vi "Read Publish Camera Settings Msg.vi"(8 "error in (no error)":errorcluster, 11 "Camera Actor in":refnum<class "Camera Actor.lvclass">) -> (0 "error out":errorcluster, 2 "Camera Actor.lvlib:Publish Camera Settings Msg.lvclass":refnum<class "Publish Camera Settings Msg.lvclass">, 3 "Camera Actor out":refnum<class "Camera Actor.lvclass">)   [LabVIEW 2020, in "Camera Actor.lvlib" / "Camera Actor.lvclass"]
uses:
  Camera Actor.lvclass
  Camera Actor Messages/Publish Camera Settings Msg/Publish Camera Settings Msg.lvclass
  Camera Actor.lvclass/Camera Actor.ctl
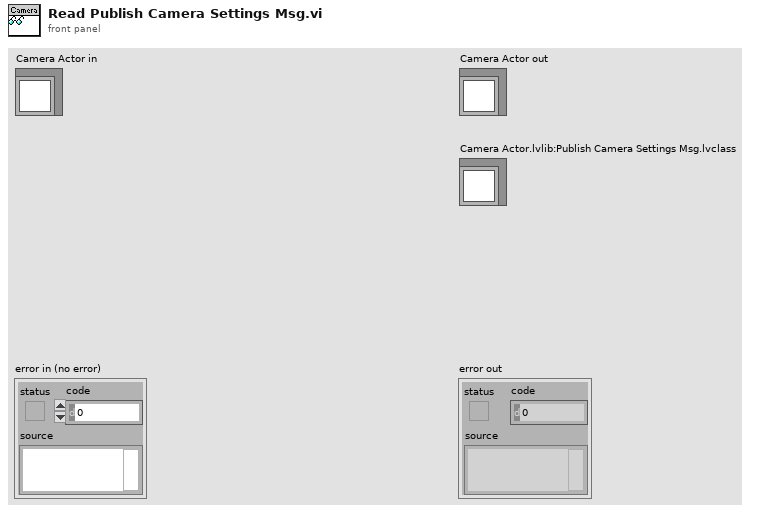
[diagram p1: front panel]
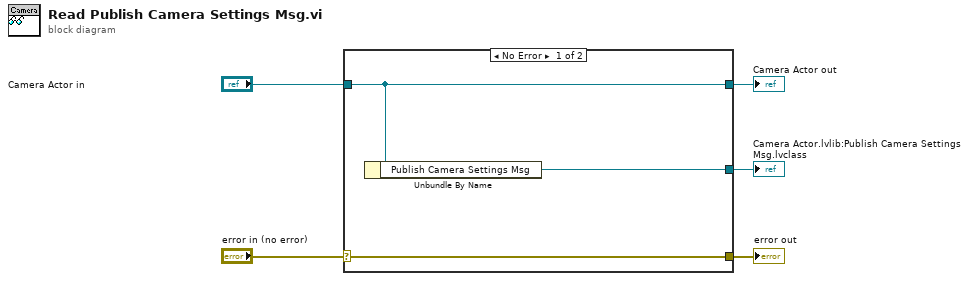
[diagram p0: block diagram]
diagram:
  n1 = case shown="No Error" "error in (no error)" {
    selector: "error in (no error)" -> [w8 w9]
    tunnel: [w8 w9] -> w4
    tunnel: [w7 w10] -> w2
    tunnel: "Camera Actor in" -> [w7 w10]
    tunnel: [w6 _] -> w1
    frame No Error {
      n2 = Unbundle By Name(w7) -> ("Publish Camera Settings Msg"=w6:refnum<class "Publish Camera Settings Msg.lvclass">)
    }
    frame Error {
    }
  }
  "error out" <- w4
  "Camera Actor out" <- w2
  "Camera Actor.lvlib:Publish Camera Settings Msg.lvclass" <- w1
